vi "Load Help File.vi"(8 "error in (no error)":errorcluster, 9 "HTML File to Load":string="MainPage_J1939.html", 10 "Main CHM File":string="J1939.chm", 11 "Browser":refnum<k7>(container)) -> (0 "error out":errorcluster, 3 "concatenated string":string)   [LabVIEW 2020, in "AIM ARINC 664 System Explorer.lvlib" / "Implementation.lvlib"]
doc: "Loads the specified HTML page from the CHM into the browser"
uses:
  Implementation.lvlib
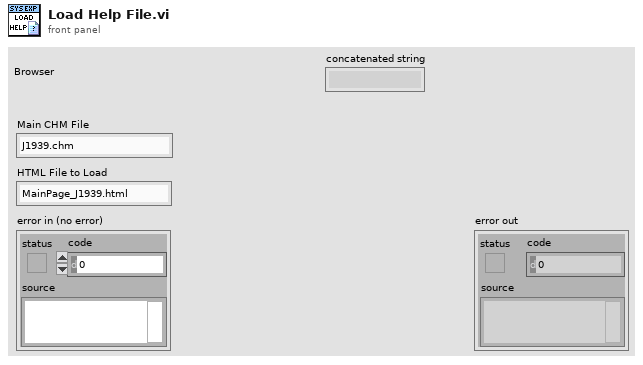
[diagram p1: front panel]
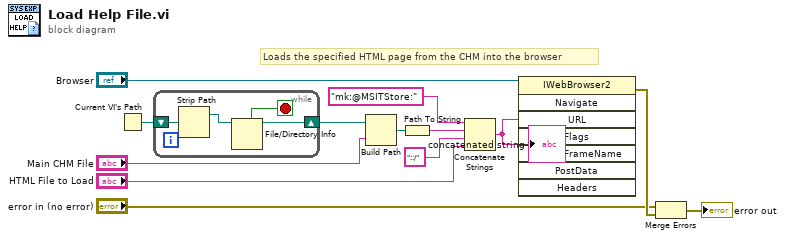
[diagram p0: block diagram]
diagram:
  # "Loads the specified HTML page from the CHM into the browser"
  n1 = Current VI's Path() -> (path=w12:path)
  n2 = while {
    shift-right: [w15] -> w3
    shift-left: w12 -> [w17]
    stop <- w14 stop-if-true
    n3 = Strip Path(path=w17) -> (stripped path=w16:path)  [unwired: 1 out]
    n4 = File/Directory Info(path=w16) -> (path out=w15:path, directory=w14:bool)  [unwired: 1 in, 5 out]
  }
  n5 = Build Path(base path=w3, name or relative path="Main CHM File") -> (appended path=w10:path)
  n6 = Path To String(path=w10) -> (string=w2:string)
  n7 = Concatenate Strings("mk:@MSITStore:" ("string"), w2, "::/" ("name or relative path"), "HTML File to Load") -> (w1:string)
  "concatenated string" <- w1
  n8 = invoke class="IWebBrowser2" method="Navigate"(reference="Browser", "URL"=w1) -> (error out=w6:errorcluster)  [unwired: 6 in, 7 out]
  n9 = Merge Errors("error in (no error)", w6) -> (→"error out":errorcluster)
